vi "LVClass_CorrectionDataManager GetDeltaCommandsFromDeltaSlopes.vi"(0 "CorrectionDataManager in":refnum<class "CorrectionDataManager.lvclass">, 5 "Delta Slopes IN":refnum<class "HasoSlopes.lvclass">, 11 "error in (no error)":errorcluster) -> (4 "CorrectionDataManager out":refnum<class "CorrectionDataManager.lvclass">, 6 "Delta Slope OUT":refnum<class "HasoSlopes.lvclass">, 8 "Mirror preferences":T2, 10 "DeltaPosition":T1, 15 "error out":errorcluster)   [LabVIEW 2020, in "CorrectionDataManager.lvclass"]
doc: "--------------------------------------------------------------------------------\n\n<B>corrdata_managerIn</B> : CorrDataManager object.\n\n<B>corrdata_managerOut</B> : CorrDataManager object.\n\n<B>delta_slopes</B> : Array of target slopes deltas (stored as cHasoSlopes).\n\n<B>gain</B> : Smoothing factor for loop iterations.\n\n<B>delta_Commands</B> : Array of size actuators count, containing the commands deltas (relatives\n variations to apply from actuators initial positions).\n\n<B>min</B> : WavefrontCorrector preferences : lowest command value.\n\n<B>max</B> : WavefrontCorrector preferences : highest command value.\n\n<B>validity</B> : WavefrontCorrector preferences : status.\n\n<B>fixed_values</B> : WavefrontCorrector preferences : fixed positions.\n\n<B>ErrorIn</B> : Error\n\n<B>ErrorOut</B> : Error"
uses:
  CorrectionDataManager.lvclass
  HasoSlopes.lvclass
  Wavefront Corrector states.ctl
  Wavefront Corrector states - ONE.ctl
  Wavefront Corrector Position.ctl
  CorrectionDataManager.lvclass/CorrectionDataManager.ctl
  LVClass_HasoSlopes Read HasoSlopes _ property.vi
panel:
  # "WavefrontCorrectorOffsetState not be used"
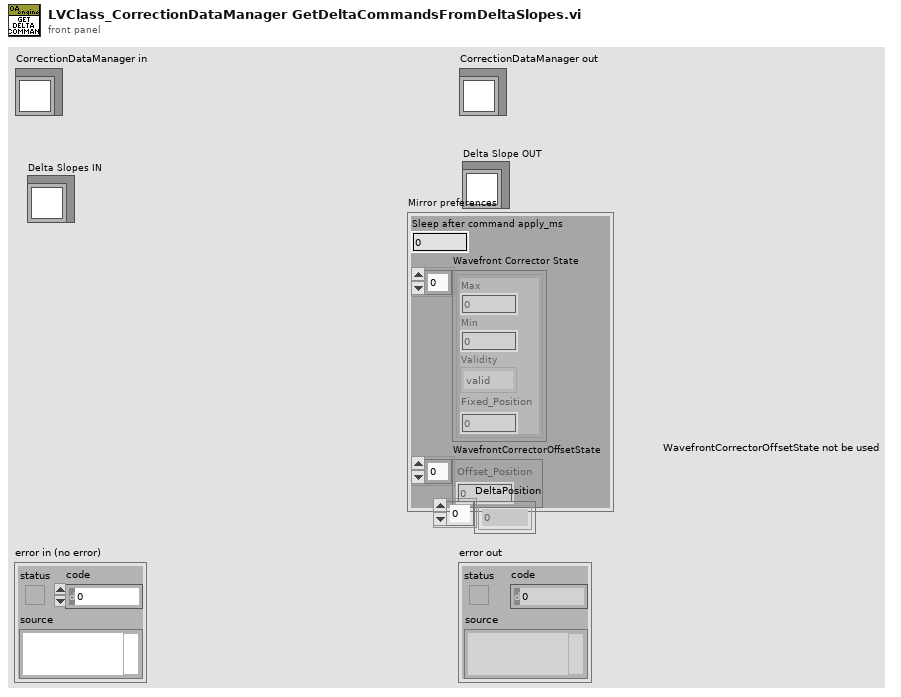
[diagram p1: front panel]
types:
  T1 = typedef "Wavefront Corrector Position.ctl" = sgl[]
  T2 = typedef "Wavefront Corrector states.ctl" = cluster{"Sleep after command apply_ms":i32, "Wavefront Corrector State":T3[], "WavefrontCorrectorOffsetState":sgl[]}
  T3 = typedef "Wavefront Corrector states - ONE.ctl" = cluster{"Max":sgl, "Min":sgl, "Validity":enum16{"valid", "fixed", "invalid"}, "Fixed_Position":sgl}
  T4 = cluster{"Sleep after command apply_ms":i32, "Wavefront Corrector State":T3[], sgl[]}
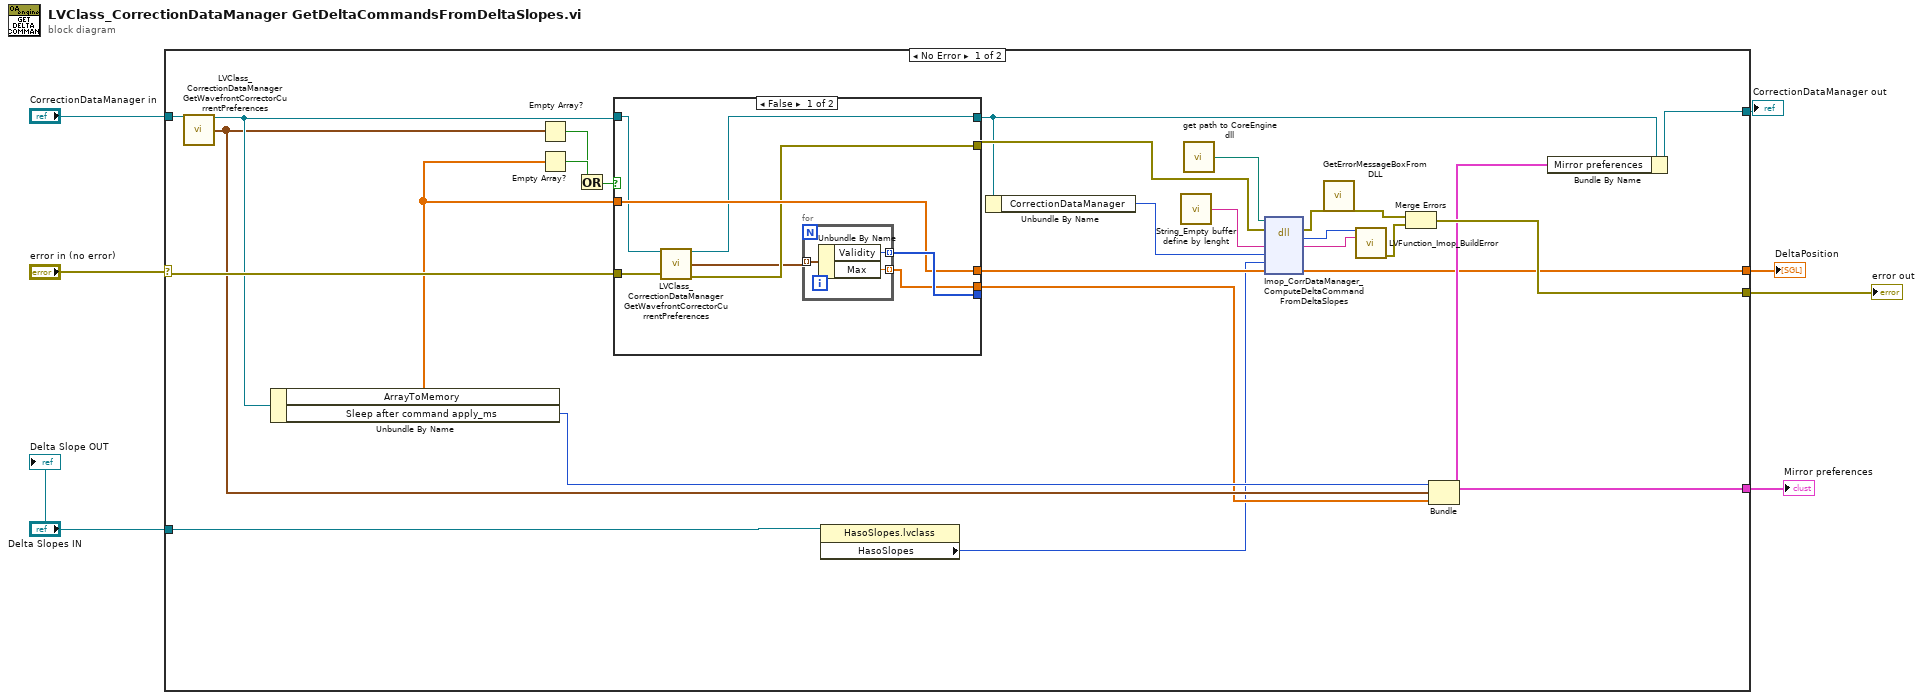
[diagram p0: block diagram]
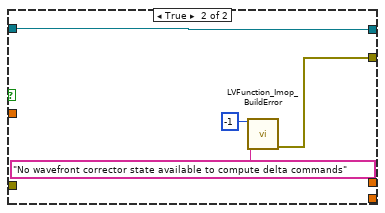
[diagram p2: hidden frame]
diagram:
  n1 = case shown="No Error" "error in (no error)" {
    selector: "error in (no error)" -> [w26 w51]
    tunnel: [w27 w51] -> w7
    tunnel: [w23 w50] -> w6
    tunnel: "CorrectionDataManager in" -> [w14 w50]
    tunnel: "Delta Slopes IN" -> [w9 _]
    tunnel: [w22 _] -> w2
    tunnel: [w11 _] -> w1
    frame No Error {
      n2 = call "LVClass_CorrectionDataManager GetWavefrontCorrectorCurrentPreferences.vi"("CorrectionDataManager in"=w14) -> ("CorrectionDataManager out"=w13:refnum<class "CorrectionDataManager.lvclass">, "Wavefront Corrector State"=w12:T3[])  [unwired: 12 in, 1 out]
      n3 = Unbundle By Name(w13) -> ("ArrayToMemory"=w15:T1, "Sleep after command apply_ms"=w21:i32)
      n4 = Empty Array?(array=w12) -> (empty?=w18:bool)
      n5 = Empty Array?(array=w15) -> (empty?=w19:bool)
      n6 = Or(x=w19, y=w18) -> (x .or. y?=w17:bool)
      n7 = case shown="False" w17 {
        tunnel: w13 -> [w36 w49]
        tunnel: [w35 w49] -> w24
        tunnel: [w41 _] -> w10
        tunnel: [w42 _] -> _
        tunnel: w26 -> [w39 _]
        tunnel: [w38 w48] -> w25
        tunnel: [w40 _] -> w16
        tunnel: w15 -> [w40 _]
        frame False {
          n8 = call "LVClass_CorrectionDataManager GetWavefrontCorrectorCurrentPreferences.vi"("CorrectionDataManager in"=w36, "error in (no error)"=w39) -> ("CorrectionDataManager out"=w35:refnum<class "CorrectionDataManager.lvclass">, "Wavefront Corrector State"=w37:T3[], "error out"=w38:errorcluster)  [unwired: 11 in]
          n9 = for {
            tunnel: w37 -> [w45] mode=indexing
            tunnel: [w44] -> w42 mode=indexing
            tunnel: [w43] -> w41 mode=indexing
            n10 = Unbundle By Name(w45) -> ("Validity"=w44:enum16{"valid", "fixed", "invalid"}, "Max"=w43:sgl)
          }
        }
        frame True {
          n11 = call "LVFunction_Imop_BuildError.vi"("code"=-1, "String to Prepend to source (\"\")"="No wavefront corrector state available to compute delta commands" ("String to Prepend to source (\"\")")) -> ("error out"=w48:errorcluster)  [unwired: 13 in]
        }
      }
      n12 = property class="HasoSlopes.lvclass"(reference=w9) -> ("HasoSlopes"=w8:i32)  [unwired: 1 in, 2 out]
      n13 = Unbundle By Name(w24) -> ("CorrectionDataManager"=w20:i32)
      n14 = call "String_Empty buffer define by lenght.vi"() -> ("Empty buffer"=w32:string)  [unwired: 1 in]
      n15 = call "get path to CoreEngine dll.vi"() -> ("path to c_interface_vc100.dll"=w31:path)  [unwired: 12 in, 3 out]
      n16 = dll-call lib="D:/FLE/0.Code/CoreEngine4_Suite/LV2011_interface/DLLs/c_interface_vc100.dll" fn="Imop_CorrDataManager_ComputeDeltaCommandFromDeltaSlopes"(path in=w31, error in=w25, "message"=w32, "WavefrontCorrection"=w20, "DeltaHasoSlopes"=w8, "delta_commands"=w16) -> (error out=w30:errorcluster, "return type"=w34:i32, "message"=w33:string, "delta_commands"=w11:sgl[])  [unwired: 3 in, 1 out]
      n17 = call "GetErrorMessageBoxFromDLL.vi"("error IN"=w30) -> ("error OUT"=w29:errorcluster)  [unwired: 10 in]
      n18 = call "LVFunction_Imop_BuildError.vi"("code"=w34, "String to Prepend to source (\"\")"=w33) -> ("error out"=w28:errorcluster)  [unwired: 13 in]
      n19 = Merge Errors(w29, w28) -> (w27:errorcluster)
      n20 = Bundle("Sleep after command apply_ms"=w21, "Wavefront Corrector State"=w12, w10) -> (w22:T4)  [unwired: 1 in]
      n21 = Bundle By Name(cluster=w24, "Mirror preferences"=w22) -> (w23:refnum<class "CorrectionDataManager.lvclass">)
    }
    frame Error {
    }
  }
  "error out" <- w7
  "CorrectionDataManager out" <- w6
  "Mirror preferences" <- w2
  "DeltaPosition" <- w1
  "Delta Slope OUT" <- "Delta Slopes IN"
